vi "PH_PowerUnit_BaseClass.pack PSDB Data.vi"(0 "VI in":refnum<vi>, 5 "error in (no error)":errorcluster) -> (14 "VI out":refnum<vi>, 16 "PSDB Boolean Data Array":T2[](array[typedef]), 17 "PSDB Numeric Data Array":T1[](array[typedef]), 18 "PSDB String Data Array":T3[](array[typedef]), 19 "error out":errorcluster)   [LabVIEW 2014, in "PH_PowerUnit_BaseClass.lvlib"]
doc: "This VI packs data for the PHELIX shot data base."
uses:
  PH_PowerUnit_BaseClass.lvlib
  PH_PSDBWriter/PH_PSDBWriter.String dataset.ctl
  PH_PSDBWriter/PH_PSDBWriter.Boolean dataset.ctl
  PH_PSDBWriter/PH_PSDBWriter.Numeric dataset.ctl
  PH_PowerUnit_BaseClass.SM States.ctl
  PH_PSDBWriter/PH_PSDBWriter.lvlib
  PH_StatusHandler/PH_StatusHandler.lvlib
  CS_Core/BaseSM/BaseSM.lvlib
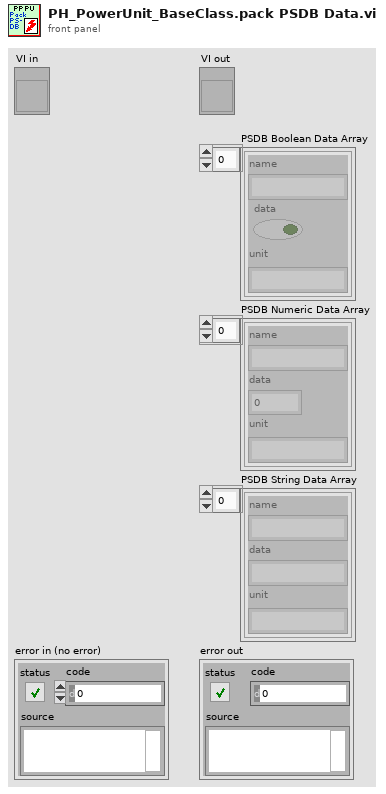
[diagram p1: front panel]
types:
  T1 = typedef "PH_PSDBWriter.lvlib/PH_PSDBWriter.Numeric dataset.ctl" = cluster{"name":string, "data":dbl, "unit":string}
  T2 = typedef "PH_PSDBWriter.lvlib/PH_PSDBWriter.Boolean dataset.ctl" = cluster{"name":string, "data":bool, "unit":string}
  T3 = typedef "PH_PSDBWriter.lvlib/PH_PSDBWriter.String dataset.ctl" = cluster{"name":string, "data":string, "unit":string}
  T4 = typedef "PH_PowerUnit_BaseClass.lvlib/PH_PowerUnit_BaseClass.i attribute.ctl" = cluster{"Constructor finished":bool, "PU":cluster{"In use":bool, "Service ID in use":i32, "GUI Ref":refnum<vi>}, "Enabling":cluster{"State":T5, "GUI Ref":refnum<vi>}, "Timing":cluster{"Last Shot":dbl, "Time between Shots [Sec]":dbl, "Waiting Time over?":bool, "Service ID Waiting Time":i32, "GUI Ref":refnum<vi>, "Instance":cluster{"Status":T6, "linked?":bool, "GUI Ref":refnum<vi>}}, "Sequencer":cluster{"SM State":string, "GUI Ref":refnum<vi>, "linked":bool}, "Subscribed Trendmssgs":cluster{"Tagname":string, "Status":T6, "linked?":bool, "Shot Condition":T6, "GUI Ref":refnum<vi>}[], "PP PU":T7, "Default Voltage (V)":dbl, "GUI Refs":T8, "PSDB data":cluster{"Shot Voltage [V]":dbl, "State TO SM":T9, "Write 2 early":bool}, "State TO SM":T9}
  T5 = typedef "PH_SystemInformation.lvlib/PH_SystemInformationEnabling State.ctl" = i32
  T6 = typedef "PH_StatusHandler.lvlib/PH_StatusHandler.Status.ctl" = i16
  T7 = typedef "PH_PP_Common.lvlib/PH_PP_Common.PUs.ctl" = enum16{"no Info", "PA-19mm-1", "PA-19mm-2", "PA-45mm-PILC", "PA-45mm-MAIN", "MA-PU-1", "MA-PU-2", "MA-PU-3", "MA-PU-4", "MA-PU-5", "MA-PU-6", "MA-FR", "MA-PILC", "PA-45mm-DP"}
  T8 = typedef "PH_PowerUnit_BaseClass.lvlib/PH_PowerUnit_BaseClass.GUI Refs.ctl" = cluster{"Delete Inst":refnum<vi>, "State TO SM":refnum<vi>, "State SM":refnum<vi>, "Fire":refnum<vi>}
  T9 = typedef "PH_PowerUnit_BaseClass.lvlib/PH_PowerUnit_BaseClass.SM States.ctl" = enum16{".", "Stand by", "Switch PU on", "Configure", "Set Default Voltage", "Set STANDBY", "Set READY", "Wait for Shot Cmd", "Open Dump Rods", "Open Ross Relais", "Close Ross Relais", "Switch PSU on", "Switch PSU off", "Charge", "Switch GD Channel on", "Close Dump Rods", "Rods-TO", "RR-TO", "PSU-TO", "Trigger-TO"}
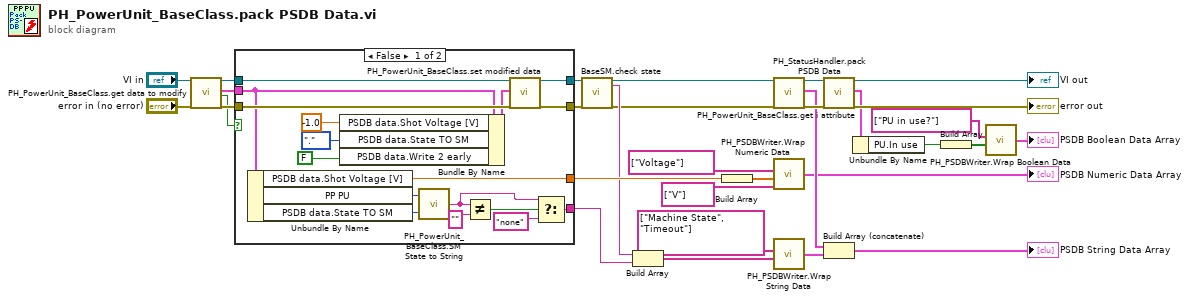
[diagram p0: block diagram]
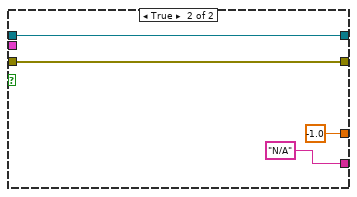
[diagram p2: hidden frame]
diagram:
  n1 = call "PH_PowerUnit_BaseClass.get data to modify.vi"("i ref in"="VI in", "error in (no error)"="error in (no error)") -> ("i ref out"=w22:refnum<vi>, "i attribute"=w20:T4, "timed out"=w19:bool, "error out"=w21:errorcluster)  [unwired: 14 in]
  n2 = case shown="False" w19 {
    tunnel: w22 -> [w48 w52]
    tunnel: w21 -> [w47 w51]
    tunnel: [w46 w52] -> w17
    tunnel: [w45 w51] -> w18
    tunnel: [w44 -1.0 ("Shot Voltage [V]")] -> w12
    tunnel: w20 -> [w43 _]
    tunnel: [w33 "N/A" ("State TO SM")] -> w13
    frame False {
      n3 = Unbundle By Name(w43) -> ("PSDB data.Shot Voltage [V]"=w44:dbl, "PP PU"=w37:T7, "PSDB data.State TO SM"=w40:T9)
      n4 = Bundle By Name(cluster=w43, "PSDB data.Shot Voltage [V]"=-1.0, "PSDB data.State TO SM"=PH_PowerUnit_BaseClass.SM_States.".", "PSDB data.Write 2 early"=FALSE) -> (w42:T4)
      n5 = call "PH_PowerUnit_BaseClass.SM State to String.vi"("SM State"=w40, "PU"=w37) -> ("SM State String"=w34:string)
      n6 = Not Equal?(x=w34, y="") -> (x != y?=w35:bool)
      n7 = call "PH_PowerUnit_BaseClass.set modified data.vi"("i ref in"=w48, "i attribute"=w42, "error in (no error)"=w47) -> ("i ref out"=w46:refnum<vi>, "error out"=w45:errorcluster)  [unwired: 15 in]
      n8 = Select(t=w34, s=w35, f="none") -> (s? t:f=w33:string)
    }
    frame True {
    }
  }
  n9 = call "BaseSM.check state.vi"("i ref in"=w17, "error in (no error)"=w18) -> ("i ref out"=w9:refnum<vi>, "actualState"=w11:string, "error out"=w7:errorcluster)  [unwired: 12 in, 3 out]
  n10 = Build Array(w11, w13) -> (w14:string[])
  n11 = Build Array(w12) -> (w16:dbl[])
  n12 = call "PH_StatusHandler.pack PSDB Data.vi"("VI in"=w9, "error in (no error)"=w7) -> ("VI out"=w24:refnum<vi>, "PSDB String Data Array"=w5:T3[], "error out"=w25:errorcluster)  [unwired: 15 in]
  n13 = call "PH_PSDBWriter.Wrap Numeric Data.vi"("Unit Array"=string[] ["V"], "Data Array"=w16, "Name Array"=string[] ["Voltage"]) -> ("PSDB Numeric Data Array"=→"PSDB Numeric Data Array":T1[])  [unwired: 1 in]
  n14 = call "PH_PSDBWriter.Wrap String Data.vi"("Data Array"=w14, "Name Array"=string[] ["Machine State", "Timeout"]) -> ("PSDB String Data Array"=w6:T3[])  [unwired: 2 in]
  n15 = call "PH_PowerUnit_BaseClass.get i attribute.vi"("i ref in"=w24, "error in (no error)"=w25) -> ("i ref out"=→"VI out":refnum<vi>, "i attribute"=w26:T4, "error out"=→"error out":errorcluster)  [unwired: 15 in]
  n16 = Build Array (concatenate)(w5, w6) -> (→"PSDB String Data Array":T3[])
  n17 = Unbundle By Name(w26) -> ("PU.In use"=w29:bool)
  n18 = Build Array(w29) -> (w28:bool[])
  n19 = call "PH_PSDBWriter.Wrap Boolean Data.vi"("Data Array"=w28, "Name Array"=string[] ["PU in use?"]) -> ("PSDB Boolean Data Array"=→"PSDB Boolean Data Array":T2[])  [unwired: 2 in]
